vi "3- image processing  edit.vi"() -> ()   [LabVIEW 2016]
uses:
  <vilib>/Instr/_visa.llb/VISA Configure Serial Port (Instr).vi
  <vilib>/vision/NI_Vision_Development_Module.lvlib
panel:
  in  "Stop (F)":bool
  out "decimal integer string 2":string
  out "return count 2":u32
  out "decimal integer string":string
  out "red":dbl
  out "green":dbl
  in  "VISA resource name 3":refnum<visa-resource-name>
  out "return count":u32
  out "green":bool
  out "red":bool
  out "Color Spectrum":dbl[](array[numeric]) format="%.2f"
  out "Image Out":T1(plugin-control)
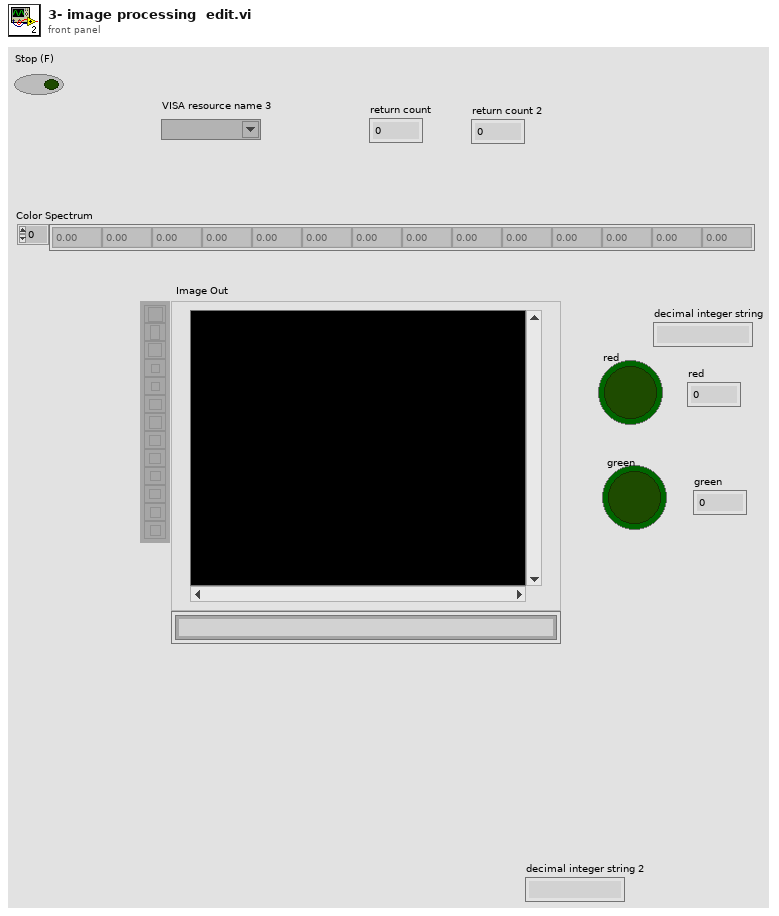
[diagram p1: front panel]
types:
  T1 = typedef "IMAQ Image.ctl" = refnum<image>
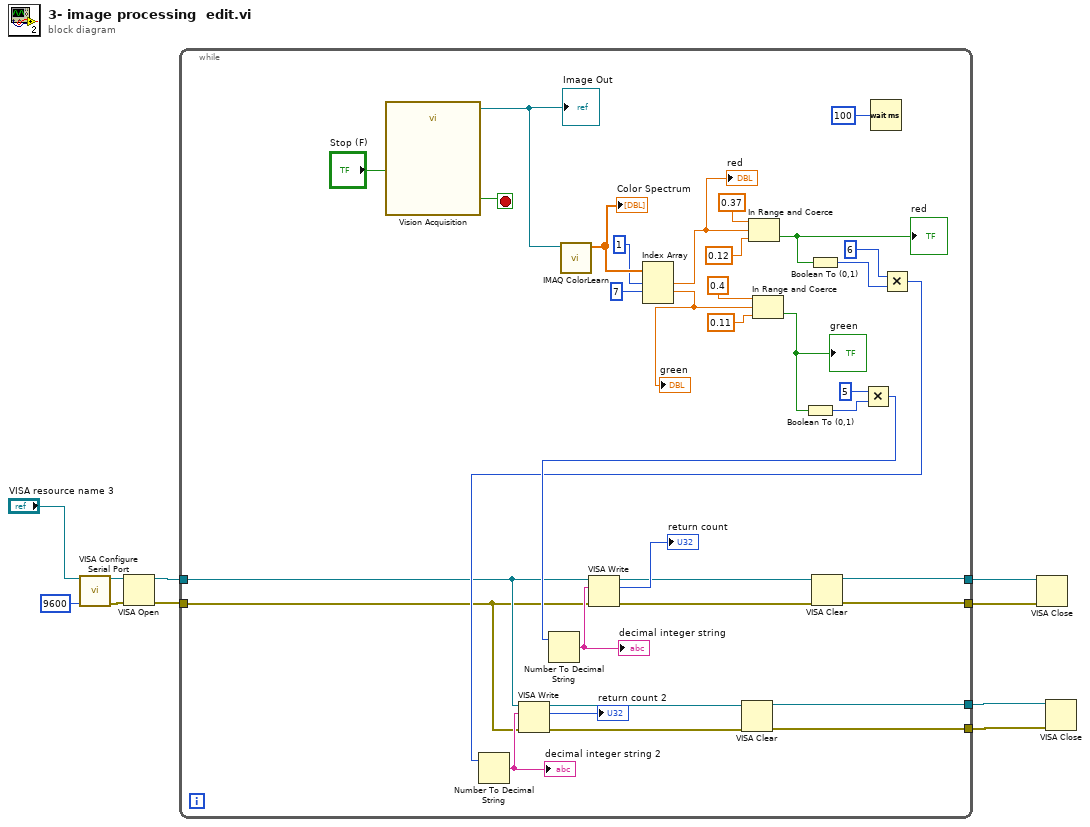
[diagram p0: block diagram]
diagram:
  n1 = call-poly "VISA Configure Serial Port"("VISA resource name"="VISA resource name 3", "baud rate (9600)"=u32 9600) -> ("VISA resource name out"=w8:refnum<visa-resource-name>, "error out"=w7:errorcluster)  [unwired: 12 in]
  n2 = VISA Open(error in (no error)=w7, VISA resource name=w8) -> (VISA resource name=w4:refnum<visa-resource-name>, error out=w3:errorcluster)  [unwired: 3 in]
  n3 = while {
    tunnel: [w25] -> w6
    tunnel: [w26] -> w5
    tunnel: w4 -> [w15]
    tunnel: w3 -> [w14]
    tunnel: [w18] -> w2
    tunnel: [w17] -> w1
    stop <- w11 stop-if-true
    n4 = call "Vision Acquisition"("Stop (F)"="Stop (F)") -> ("Image Out"=w12:T1, "Stopped"=w11:bool)  [unwired: 24 in, 1 out]
    "Image Out" <- w12
    n5 = call "IMAQ ColorLearn"("Image"=w12) -> ("Color Spectrum"=w45:dbl[])  [unwired: 7 in, 1 out]
    "Color Spectrum" <- w45
    n6 = Index Array(array=w45, index #1=1 ("index"), index #2=7 ("index")) -> (element #1=w33:dbl, element #2=w24:dbl)  [unwired: 1 in, 1 out]
    "green" <- w24
    "red" <- w33
    n7 = In Range and Coerce(upper limit=0.37, x=w33, lower limit=0.12) -> (In Range?=w29:bool)  [unwired: 1 out]
    "red" <- w29
    n8 = In Range and Coerce(upper limit=0.4, x=w24, lower limit=0.11) -> (In Range?=w32:bool)  [unwired: 1 out]
    "green" <- w32
    n9 = Boolean To (0,1)(Boolean=w32) -> (0, 1=w34:i16)
    n10 = Boolean To (0,1)(Boolean=w29) -> (0, 1=w30:i16)
    n11 = Multiply(x=i16 5, y=w34) -> (x*y=w23:i16)
    n12 = Number To Decimal String(number=w23) -> (decimal integer string=w38:string)  [unwired: 1 in]
    "decimal integer string" <- w38
    n13 = VISA Write(VISA resource name=w15, write buffer=w38, error in (no error)=w14) -> (VISA resource name out=w28:refnum<visa-resource-name>, return count=→"return count":u32, error out=w27:errorcluster)
    n14 = VISA Clear(VISA resource name=w28, error in (no error)=w27) -> (VISA resource name out=w25:refnum<visa-resource-name>, error out=w26:errorcluster)
    n15 = Wait (ms)(milliseconds to wait=u32 100 ("millisecond multiple")) -> ()  [unwired: 1 out]
    n16 = Multiply(x=i16 6, y=w30) -> (x*y=w16:i16)
    n17 = Number To Decimal String(number=w16) -> (decimal integer string=w22:string)  [unwired: 1 in]
    "decimal integer string 2" <- w22
    n18 = VISA Write(VISA resource name=w15, write buffer=w22, error in (no error)=w14) -> (VISA resource name out=w20:refnum<visa-resource-name>, return count=→"return count 2":u32, error out=w19:errorcluster)
    n19 = VISA Clear(VISA resource name=w20, error in (no error)=w19) -> (VISA resource name out=w18:refnum<visa-resource-name>, error out=w17:errorcluster)
  }
  n20 = VISA Close(VISA resource name=w6, error in (no error)=w5) -> ()  [unwired: 1 out]
  n21 = VISA Close(VISA resource name=w2, error in (no error)=w1) -> ()  [unwired: 1 out]
